vi "Create grid of bookmarks.vi"(0 "Stage current position":dbl[](array[numeric])) -> (15 "Output array":string[][](array[string]), 18 "Output string":string)   [LabVIEW 2017]
panel:
  out "z-pos":string
  in  "Create":bool
  in  "bidirectional":bool=TRUE
  in  "x-first":bool=TRUE
  in  "y-step (mm)":dbl=50.0
  in  "x-step (mm)":dbl=50.0
  in  "y-size":i32=5
  in  "x-size":i32=5
  in  "y-start":dbl
  in  "x-start":dbl
  # "Grid creator"
  # "unidirectional"
  # "y-first"
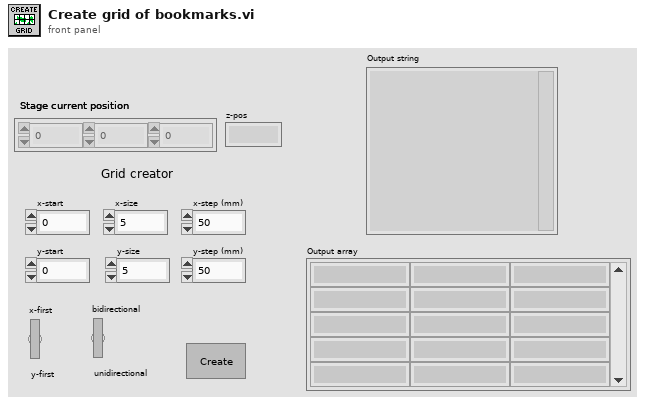
[diagram p1: front panel]
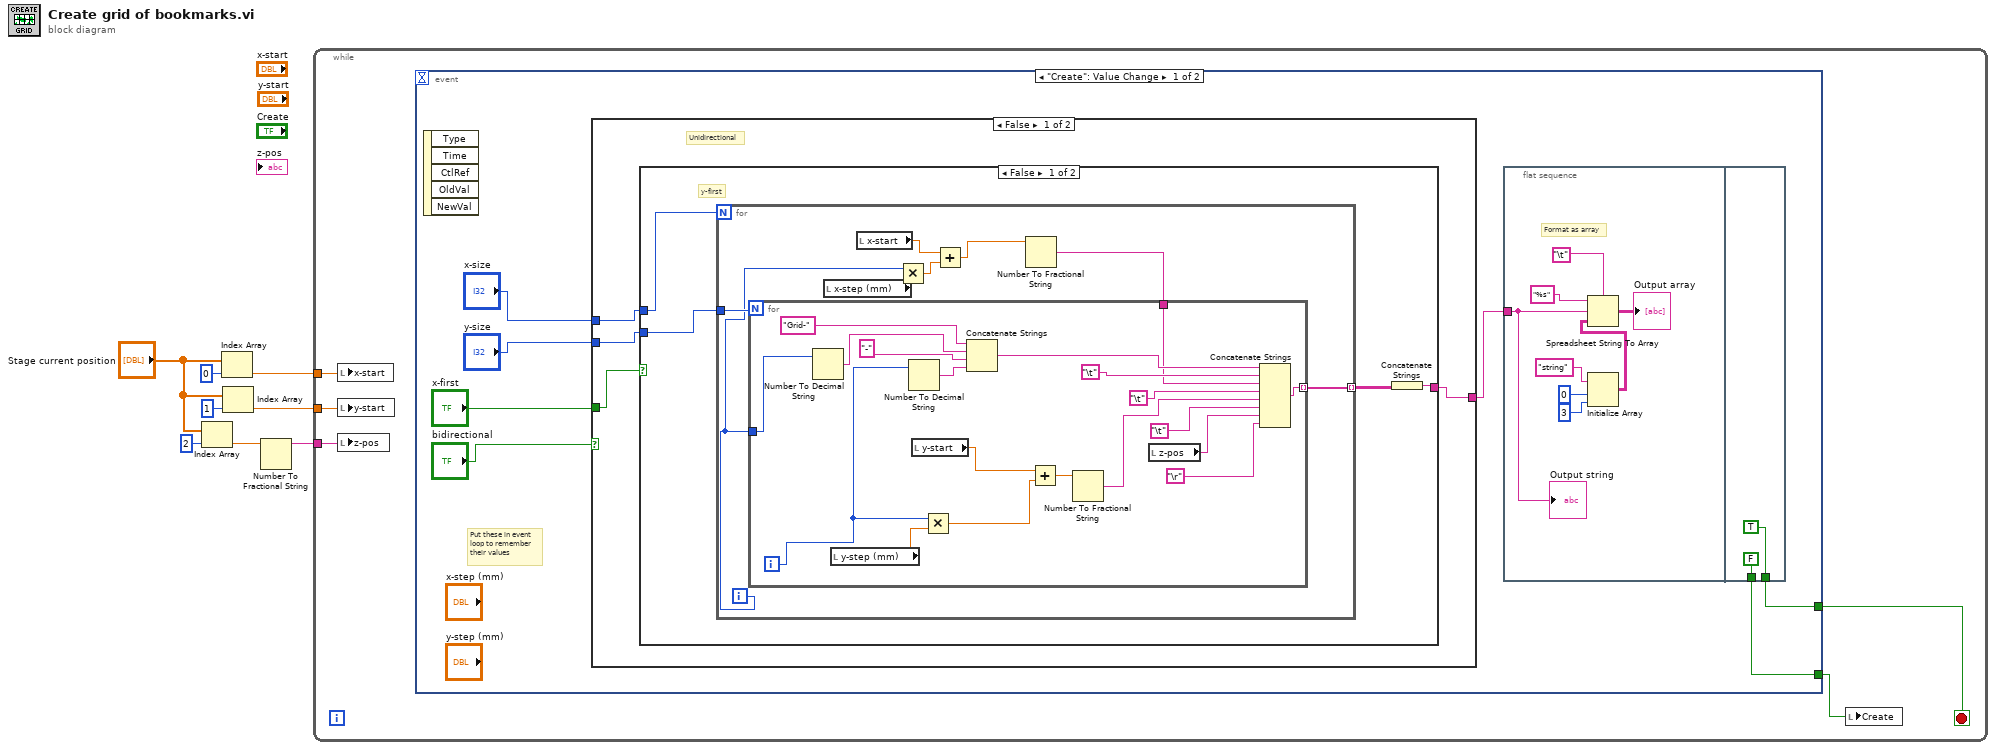
[diagram p0: block diagram]
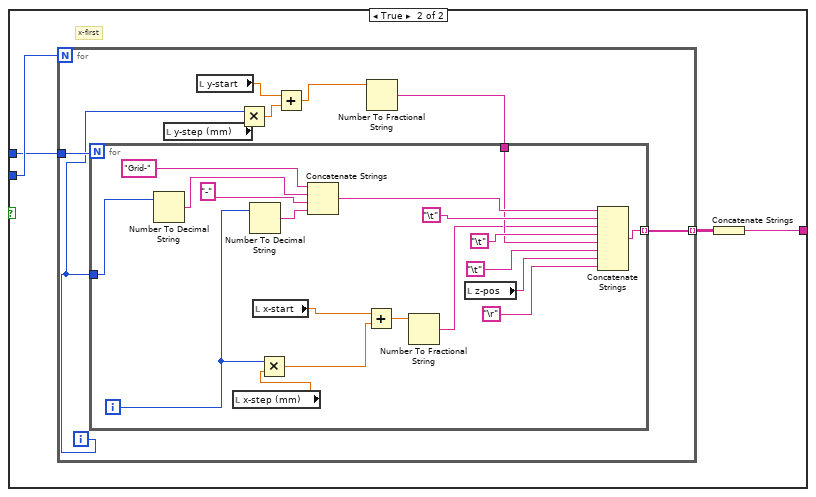
[diagram p2: hidden frame]
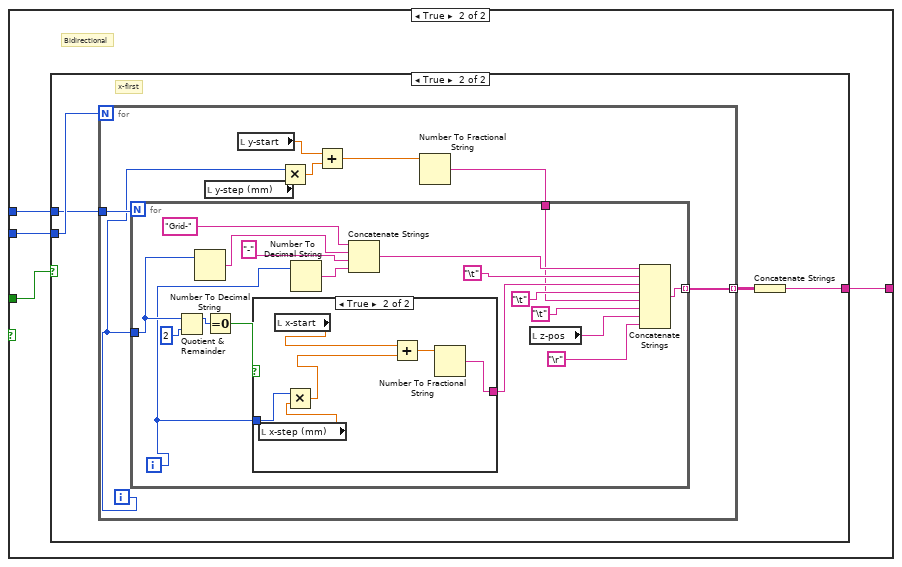
[diagram p3: hidden frame]
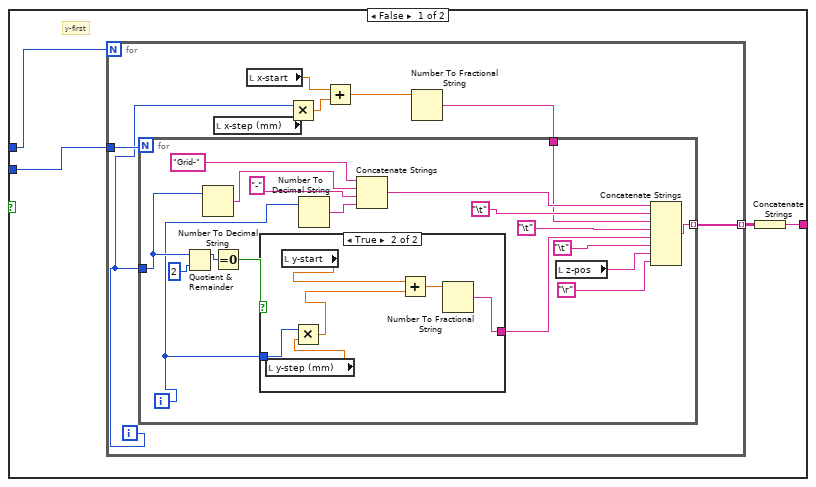
[diagram p4: hidden frame]
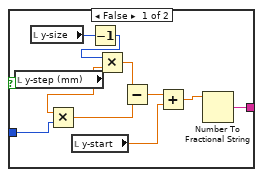
[diagram p5: hidden frame]
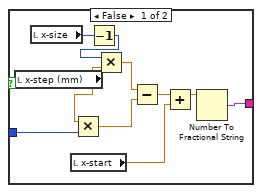
[diagram p6: hidden frame]
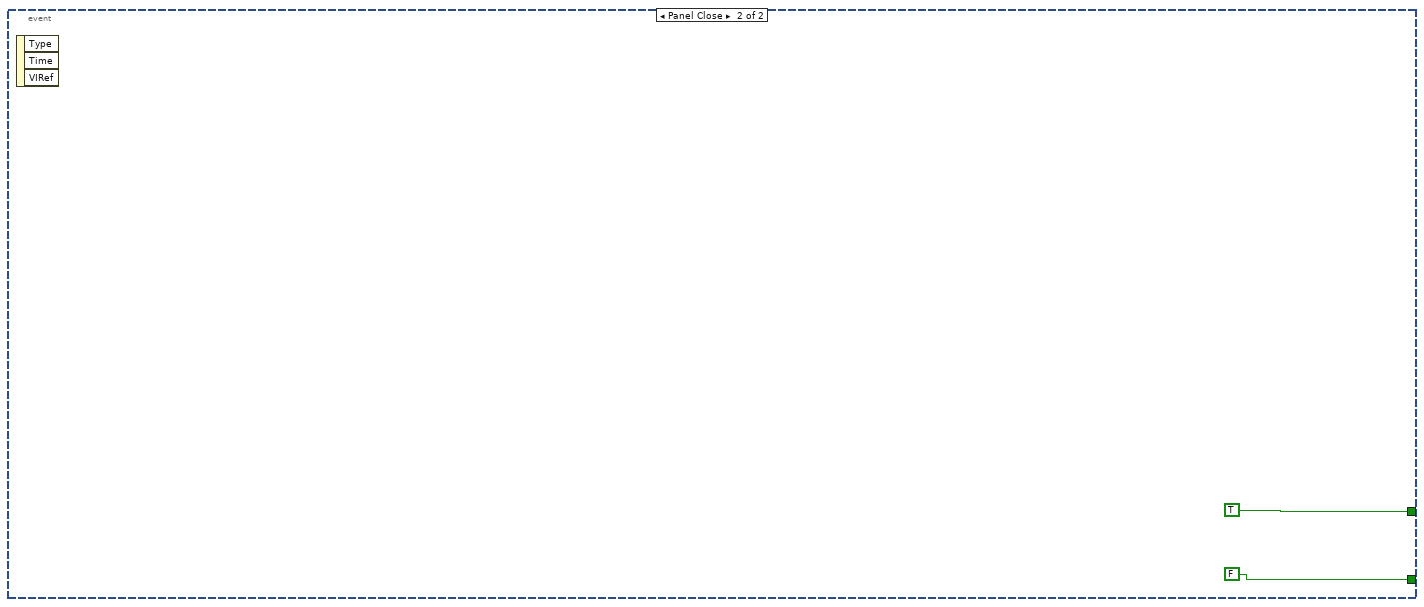
[diagram p7: hidden frame]
diagram:
  n1 = Index Array(array="Stage current position", index=2) -> (element=w2:dbl)
  n2 = Index Array(array="Stage current position", index=0) -> (element=w5:dbl)
  n3 = Index Array(array="Stage current position", index=1) -> (element=w6:dbl)
  n4 = Number To Fractional String(number=w2) -> (F-format string=w1:string)  [unwired: 3 in]
  n5 = while {
    tunnel: w6 -> [w11]
    tunnel: w5 -> [w10]
    tunnel: w1 -> [w9]
    stop <- w13 stop-if-true
    n6 = local write "x-start"(w10) -> ()
    n7 = local write "y-start"(w11) -> ()
    n8 = local write "z-pos"(w9) -> ()
    n9 = event shown="[0] \"Create\": Value Change" {
      selector: _ -> [_ _]
      dyn-events: _ -> [_ _]
      timeout: _ -> [_ _]
      tunnel: [w19 TRUE] -> w13
      tunnel: [w18 FALSE] -> w12
      event "Create": Value Change {
        # "Put these in event\nloop to remember\ntheir values"
        n10 = event-data() -> ()  [unwired: 1 in, 5 out]
        n11 = case shown="False" "bidirectional" {
          tunnel: "x-first" -> [w31 w100]
          tunnel: "y-size" -> [w33 w99]
          tunnel: "x-size" -> [w32 w98]
          tunnel: [w34 w97] -> w20
          frame False {
            # "Unidirectional"
            n12 = case shown="False" w31 {
              tunnel: w33 -> [w37 w69]
              tunnel: w32 -> [w38 w68]
              tunnel: [w35 w66] -> w34
              frame False {
                # "y-first"
                n13 = for {
                  N: w38 -> [_]
                  tunnel: w37 -> [w46]
                  tunnel: [w39] -> w36 mode=indexing
                  i -> [w44]
                  n14 = local read "x-step (mm)"() -> (w45:dbl)
                  n15 = local read "x-start"() -> (w42:dbl)
                  n16 = Multiply(x=w44, y=w45) -> (x*y=w43:dbl)
                  n17 = Add(x=w42, y=w43) -> (x+y=w41:dbl)
                  n18 = Number To Fractional String(number=w41) -> (F-format string=w40:string)  [unwired: 3 in]
                  n19 = for {
                    N: w46 -> [_]
                    tunnel: w44 -> [w65]
                    tunnel: w40 -> [w51]
                    tunnel: [w57] -> w39 mode=indexing
                    i -> [w52]
                    n20 = Number To Decimal String(number=w65) -> (decimal integer string=w63:string)  [unwired: 1 in]
                    n21 = local read "y-step (mm)"() -> (w55:dbl)
                    n22 = Number To Decimal String(number=w52) -> (decimal integer string=w61:string)  [unwired: 1 in]
                    n23 = local read "y-start"() -> (w53:dbl)
                    n24 = Multiply(x=w52, y=w55) -> (x*y=w54:dbl)
                    n25 = Concatenate Strings("Grid-", w63, "-", w61) -> (w60:string)
                    n26 = Add(x=w53, y=w54) -> (x+y=w56:dbl)
                    n27 = Number To Fractional String(number=w56) -> (F-format string=w50:string)  [unwired: 3 in]
                    n28 = local read "z-pos"() -> (w47:string)
                    n29 = Concatenate Strings(w60, "\t", w51, "\t", w50, "\t", w47, "\r") -> (w57:string)
                  }
                }
                n30 = Concatenate Strings(w36) -> (w35:string)
              }
              frame True {
                # "x-first"
                n31 = for {
                  N: w69 -> [_]
                  tunnel: w68 -> [w77]
                  tunnel: [w70] -> w67 mode=indexing
                  i -> [w75]
                  n32 = local read "y-step (mm)"() -> (w76:dbl)
                  n33 = local read "y-start"() -> (w73:dbl)
                  n34 = Multiply(x=w75, y=w76) -> (x*y=w74:dbl)
                  n35 = Add(x=w73, y=w74) -> (x+y=w72:dbl)
                  n36 = Number To Fractional String(number=w72) -> (F-format string=w71:string)  [unwired: 3 in]
                  n37 = for {
                    N: w77 -> [_]
                    tunnel: w75 -> [w96]
                    tunnel: w71 -> [w88]
                    tunnel: [w87] -> w70 mode=indexing
                    i -> [w83]
                    n38 = Number To Decimal String(number=w96) -> (decimal integer string=w94:string)  [unwired: 1 in]
                    n39 = local read "x-step (mm)"() -> (w82:dbl)
                    n40 = Number To Decimal String(number=w83) -> (decimal integer string=w92:string)  [unwired: 1 in]
                    n41 = local read "x-start"() -> (w81:dbl)
                    n42 = Multiply(x=w83, y=w82) -> (x*y=w85:dbl)
                    n43 = Concatenate Strings("Grid-", w94, "-", w92) -> (w91:string)
                    n44 = Add(x=w81, y=w85) -> (x+y=w86:dbl)
                    n45 = Number To Fractional String(number=w86) -> (F-format string=w84:string)  [unwired: 3 in]
                    n46 = local read "z-pos"() -> (w78:string)
                    n47 = Concatenate Strings(w91, "\t", w84, "\t", w88, "\t", w78, "\r") -> (w87:string)
                  }
                }
                n48 = Concatenate Strings(w67) -> (w66:string)
              }
            }
          }
          frame True {
            # "Bidirectional"
            n49 = case shown="True" w100 {
              tunnel: w99 -> [w103 w150]
              tunnel: w98 -> [w104 w149]
              tunnel: [w101 w147] -> w97
              frame False {
                # "y-first"
                n50 = for {
                  N: w104 -> [_]
                  tunnel: w103 -> [w112]
                  tunnel: [w105] -> w102 mode=indexing
                  i -> [w110]
                  n51 = local read "x-step (mm)"() -> (w111:dbl)
                  n52 = local read "x-start"() -> (w108:dbl)
                  n53 = Multiply(x=w110, y=w111) -> (x*y=w109:dbl)
                  n54 = Add(x=w108, y=w109) -> (x+y=w107:dbl)
                  n55 = Number To Fractional String(number=w107) -> (F-format string=w106:string)  [unwired: 3 in]
                  n56 = for {
                    N: w112 -> [_]
                    tunnel: w110 -> [w130]
                    tunnel: w106 -> [w117]
                    tunnel: [w118] -> w105 mode=indexing
                    i -> [w126]
                    n57 = Quotient & Remainder(x=w130, y=2) -> (x-y*floor(x/y)=w128:i32)  [unwired: 1 out]
                    n58 = Number To Decimal String(number=w130) -> (decimal integer string=w124:string)  [unwired: 1 in]
                    n59 = Equal To 0?(x=w128) -> (x = 0?=w127:bool)
                    n60 = case shown="True" w127 {
                      tunnel: w126 -> [w138 w143]
                      tunnel: [w134 w141] -> w116
                      frame False {
                        n61 = local read "y-step (mm)"() -> (w137:dbl)
                        n62 = local read "y-size"() -> (w140:i32)
                        n63 = Multiply(x=w137, y=w138) -> (x*y=w135:dbl)
                        n64 = local read "y-start"() -> (w131:dbl)
                        n65 = Decrement(x=w140) -> (x-1=w139:i32)
                        n66 = Multiply(x=w139, y=w137) -> (x*y=w136:dbl)
                        n67 = Subtract(x=w136, y=w135) -> (x-y=w133:dbl)
                        n68 = Add(x=w133, y=w131) -> (x+y=w132:dbl)
                        n69 = Number To Fractional String(number=w132) -> (F-format string=w134:string)  [unwired: 3 in]
                      }
                      frame True {
                        n70 = local read "y-step (mm)"() -> (w144:dbl)
                        n71 = local read "y-start"() -> (w146:dbl)
                        n72 = Multiply(x=w143, y=w144) -> (x*y=w145:dbl)
                        n73 = Add(x=w146, y=w145) -> (x+y=w142:dbl)
                        n74 = Number To Fractional String(number=w142) -> (F-format string=w141:string)  [unwired: 3 in]
                      }
                    }
                    n75 = Number To Decimal String(number=w126) -> (decimal integer string=w122:string)  [unwired: 1 in]
                    n76 = Concatenate Strings("Grid-", w124, "-", w122) -> (w121:string)
                    n77 = local read "z-pos"() -> (w114:string)
                    n78 = Concatenate Strings(w121, "\t", w117, "\t", w116, "\t", w114, "\r") -> (w118:string)
                  }
                }
                n79 = Concatenate Strings(w102) -> (w101:string)
              }
              frame True {
                # "x-first"
                n80 = for {
                  N: w150 -> [_]
                  tunnel: w149 -> [w158]
                  tunnel: [w151] -> w148 mode=indexing
                  i -> [w156]
                  n81 = local read "y-step (mm)"() -> (w157:dbl)
                  n82 = local read "y-start"() -> (w154:dbl)
                  n83 = Multiply(x=w156, y=w157) -> (x*y=w155:dbl)
                  n84 = Add(x=w154, y=w155) -> (x+y=w153:dbl)
                  n85 = Number To Fractional String(number=w153) -> (F-format string=w152:string)  [unwired: 3 in]
                  n86 = for {
                    N: w158 -> [_]
                    tunnel: w156 -> [w176]
                    tunnel: w152 -> [w163]
                    tunnel: [w162] -> w151 mode=indexing
                    i -> [w172]
                    n87 = Quotient & Remainder(x=w176, y=2) -> (x-y*floor(x/y)=w174:i32)  [unwired: 1 out]
                    n88 = Number To Decimal String(number=w176) -> (decimal integer string=w170:string)  [unwired: 1 in]
                    n89 = Equal To 0?(x=w174) -> (x = 0?=w173:bool)
                    n90 = case shown="True" w173 {
                      tunnel: w172 -> [w184 w189]
                      tunnel: [w180 w187] -> w165
                      frame False {
                        n91 = local read "x-step (mm)"() -> (w183:dbl)
                        n92 = local read "x-size"() -> (w186:i32)
                        n93 = local read "x-start"() -> (w177:dbl)
                        n94 = Multiply(x=w183, y=w184) -> (x*y=w181:dbl)
                        n95 = Decrement(x=w186) -> (x-1=w185:i32)
                        n96 = Multiply(x=w185, y=w183) -> (x*y=w182:dbl)
                        n97 = Subtract(x=w182, y=w181) -> (x-y=w178:dbl)
                        n98 = Add(x=w178, y=w177) -> (x+y=w179:dbl)
                        n99 = Number To Fractional String(number=w179) -> (F-format string=w180:string)  [unwired: 3 in]
                      }
                      frame True {
                        n100 = local read "x-step (mm)"() -> (w190:dbl)
                        n101 = local read "x-start"() -> (w192:dbl)
                        n102 = Multiply(x=w189, y=w190) -> (x*y=w191:dbl)
                        n103 = Add(x=w192, y=w191) -> (x+y=w188:dbl)
                        n104 = Number To Fractional String(number=w188) -> (F-format string=w187:string)  [unwired: 3 in]
                      }
                    }
                    n105 = Number To Decimal String(number=w172) -> (decimal integer string=w168:string)  [unwired: 1 in]
                    n106 = Concatenate Strings("Grid-", w170, "-", w168) -> (w167:string)
                    n107 = local read "z-pos"() -> (w160:string)
                    n108 = Concatenate Strings(w167, "\t", w165, "\t", w163, "\t", w160, "\r") -> (w162:string)
                  }
                }
                n109 = Concatenate Strings(w148) -> (w147:string)
              }
            }
          }
        }
        n110 = flat-sequence {
          tunnel: w20 -> [w21]
          tunnel: [TRUE] -> w19
          tunnel: [FALSE] -> w18
          frame #0 {
            # "Format as array"
            n111 = Initialize Array("string" ("format string"), 0 ("dimension size"), 3 ("dimension size")) -> (w25:string[][])
            n112 = Spreadsheet String To Array(delimiter (Tab)="\t", format string="%s", spreadsheet string=w21, array type (2D Dbl)=w25) -> (array=→"Output array":string[][])
            "Output string" <- w21
          }
          frame #1 {
          }
        }
      }
      event Panel Close {
        n113 = event-data() -> ()  [unwired: 1 in, 3 out]
      }
    }
    n114 = local write "Create"(w12) -> ()
  }
